vi "U32 info.vi"(8 "error in (no error)":errorcluster, 11 "Variant":variant) -> (0 "error out":errorcluster, 3 "child strings":string[](array[string]))   [LabVIEW 2017, in "DSF Mini Explorer.lvlib"]
uses:
  DSF Configuration.llb/DSF Mini Explorer.lvlib
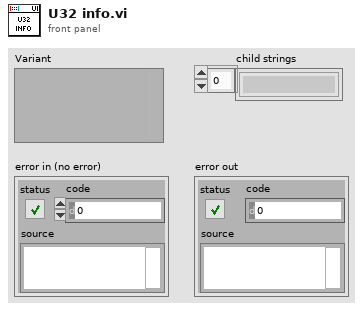
[diagram p1: front panel]
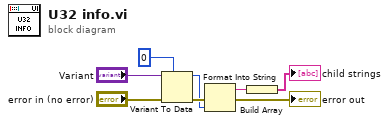
[diagram p0: block diagram]
diagram:
  n1 = Variant To Data(error in="error in (no error)", type=u32 0, Variant="Variant") -> (data=w3:u32, error out=w7:errorcluster)
  n2 = Format Into String(error in=w7, w3) -> (resulting string=w5:string, error out=→"error out":errorcluster)  [unwired: 2 in]
  n3 = Build Array(w5) -> (→"child strings":string[])
